vi "myRIO_BRig_RT_comm_webdav_hostFolder_store.vi"() -> (2 "output_HostFolder":string="myRIO_transfers")   [LabVIEW 2014]
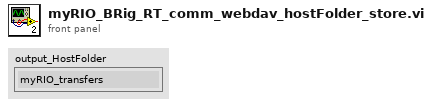
[diagram p1: front panel]
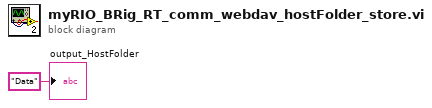
[diagram p0: block diagram]
diagram:
  "output_HostFolder" <- "Data" ("host uri prefix")
